vi "RandomDouble.vi"(10 "Min":dbl, 11 "Max":dbl) -> (3 "Random":dbl)   [LabVIEW 2009]
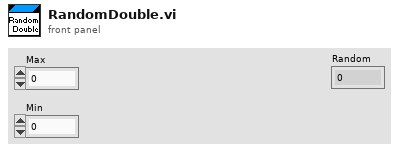
[diagram p1: front panel]
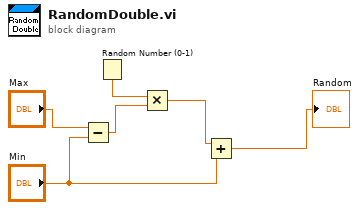
[diagram p0: block diagram]
diagram:
  n1 = Subtract(x="Max", y="Min") -> (x-y=w4:dbl)
  n2 = Random Number (0-1)() -> (number: 0 to 1=w3:dbl)
  n3 = Multiply(x=w3, y=w4) -> (x*y=w2:dbl)
  n4 = Add(x=w2, y="Min") -> (x+y=→"Random":dbl)
